vi "5900PRQuickSet.vi"(0 "VISA resource name":refnum<visa-resource-name>="GPIB::1", 1 "Panametrics Settings":T1={"ENERGY (uJ)"=0, "DAMPING (Ohm)"=0, "HP FILT (KHz) "=1, "LP FILT (MHz)"=0, "MODE"=0, "PRF (KHz)"=0, "GAIN (db)"=0, "COARSE ATTENUATION"=0, "FINE ATTENUATION"=0} {"FINE ATTENUATION" items=["00.0", "00.5", "01.0", "01.5", "02.0", "02.5", "03.0", "03.5", "04.0", "04.5", "05.0", "05.5", "06.0", "06.5", "07.0", "07.5", "08.0", "08.5", "09.0", "09.5", "10.0", "10.5", "11.0", "11.5", "12.0", "12.5", "13.0", "13.5", "14.0", "14.5", "15.0", "15.5"]; "COARSE ATTENUATION" items=["00.0", "10.0", "20.0", "30.0", "40.0", "50.0"]; "GAIN (db)" items=["26.0", "40.0", "54.0"]; "PRF (KHz)" items=["XREMT", "EXBNC", "0.200", "0.500", "1.000", "2.000", "5.000", "10.00", "20.00"]; "MODE" items=["P/ E", "THRU", "RPP", "EXT_PLSR"]; "LP FILT (MHz)" items=["20", "50", "100", "200"]; "HP FILT (KHz)" items=["1", "1000", "3000", "10000"]; "DAMPING (Ohm)" items=["7", "10", "16", "20", "26", "30", "40", "50"]; "ENERGY (uJ)" items=["1", "2", "4", "8", "16", "32"]}) -> (4 "error out":errorcluster)   [LabVIEW 2022 SP3]
uses:
  Pana5900.ctl
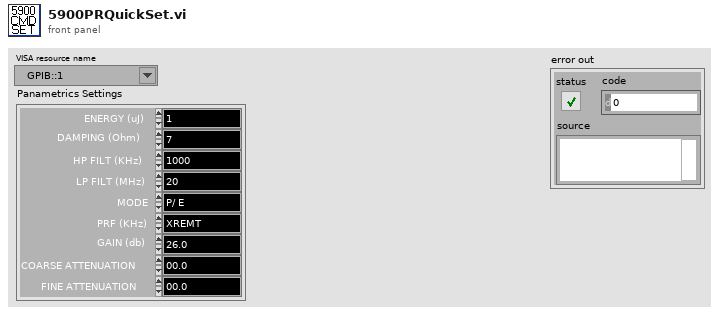
[diagram p1: front panel]
types:
  T1 = typedef "Pana5900.ctl" = cluster{"ENERGY (uJ)":u16, "DAMPING (Ohm)":u16, "HP FILT (KHz) ":u16, "LP FILT (MHz)":u16, "MODE":u16, "PRF (KHz)":u16, "GAIN (db)":u16, "COARSE ATTENUATION":u16, "FINE ATTENUATION":u16}
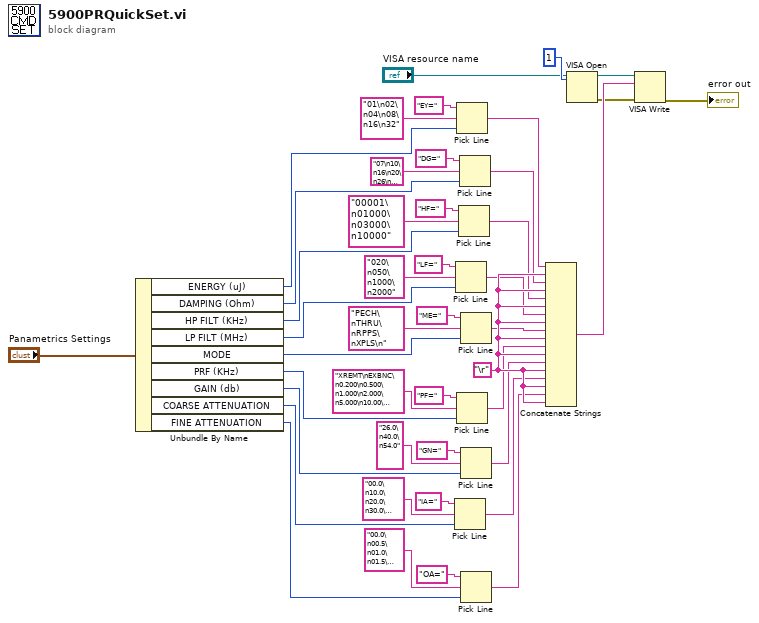
[diagram p0: block diagram]
diagram:
  w13 = "\r"
  n1 = Unbundle By Name("Panametrics Settings") -> ("ENERGY (uJ)"=w28:u16, "DAMPING (Ohm)"=w25:u16, "HP FILT (KHz)"=w22:u16, "LP FILT (MHz)"=w37:u16, "MODE"=w34:u16, "PRF (KHz)"=w31:u16, "GAIN (db)"=w14:u16, "COARSE ATTENUATION"=w19:u16, "FINE ATTENUATION"=w3:u16)
  n2 = Pick Line(string ("")="IA=", multi-line string="00.0\n10.0\n20.0\n30.0\n40.0\n50.0\n60.0", line index=w19) -> (output string=w5:string)
  n3 = Pick Line(string ("")="LF=", multi-line string="020\n050\n1000\n2000", line index=w37) -> (output string=w9:string)
  n4 = Pick Line(string ("")="EY=", multi-line string="01\n02\n04\n08\n16\n32", line index=w28) -> (output string=w12:string)
  n5 = Pick Line(string ("")="PF=", multi-line string="XREMT\nEXBNC\n0.200\n0.500\n1.000\n2.000\n5.000\n10.00\n20.00\n", line index=w31) -> (output string=w7:string)
  n6 = Pick Line(string ("")="HF=", multi-line string="00001\n01000\n03000\n10000", line index=w22) -> (output string=w10:string)
  n7 = Pick Line(string ("")="DG=", multi-line string="07\n10\n16\n20\n26\n30\n40\n50\n", line index=w25) -> (output string=w11:string)
  n8 = Pick Line(string ("")="ME=", multi-line string="PECH\nTHRU\nRPPS\nXPLS\n", line index=w34) -> (output string=w8:string)
  n9 = Pick Line(string ("")="GN=", multi-line string="26.0\n40.0\n54.0", line index=w14) -> (output string=w6:string)
  n10 = Pick Line(string ("")="OA=", multi-line string="00.0\n00.5\n01.0\n01.5\n02.0\n02.5\n03.0\n03.5\n04.0\n04.5\n05.0\n05.5\n06.0\n06.5\n07.0\n07.5\n08.0\n08.5\n09.0\n09.5\n10.0\n10.5\n11.0\n11.5\n12.0\n12.5\n13.0\n13.5\n14.0\n14.5\n15.0\n15.5", line index=w3) -> (output string=w4:string)
  n11 = Concatenate Strings(w12, w13, w11, w13, w10, w13, w9, w13, w8, w13, w7, w13, w6, w13, w5, w13, w4, w13) -> (w40:string)
  n12 = VISA Open(timeout (0)=1, VISA resource name="VISA resource name") -> (VISA resource name=w41:refnum<visa-resource-name>, error out=w2:errorcluster)  [unwired: 1 in, 2 out]
  n13 = VISA Write(VISA resource name=w41, write buffer=w40, error in (no error)=w2) -> (error out=→"error out":errorcluster)  [unwired: 2 out]
